vi "sub_register-event-callback.vi"(7 "cmd":enum16{"register", "close"}(ring), 8 "error in":errorcluster, 10 "user param":refnum<vi>[](array[refnum]), 11 "GMapControl":refnum<k24>) -> (0 "error out":errorcluster)   [LabVIEW 2019]
uses:
  dll/GMap.NET.WindowsForms.dll
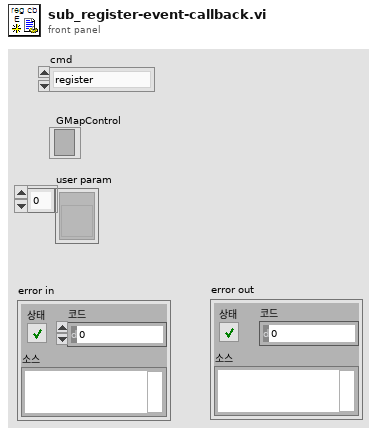
[diagram p1: front panel]
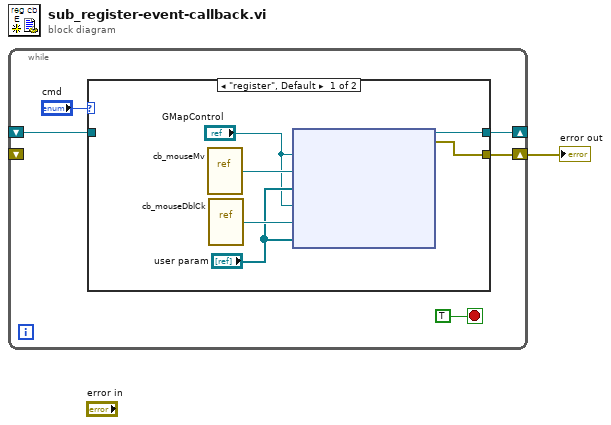
[diagram p0: block diagram]
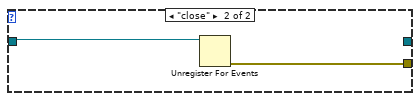
[diagram p2: hidden frame]
diagram:
  n1 = while {
    shift-right: [w3] -> _
    shift-left: _ -> [w4]
    shift-right: [w2] -> w1
    shift-left: _ -> [_]
    stop <- TRUE stop-if-true
    n2 = case shown="\"register\", Default" "cmd" {
      tunnel: w4 -> [_ w14]
      tunnel: [w10 _] -> w3
      tunnel: [w8 w13] -> w2
      frame "register", Default {
        n3 = vi-ref "cb_mouseMv.vi"() -> ("vi reference"=w12:refnum<vi>)
        n4 = vi-ref "cb_mouseDblCk.vi"() -> ("vi reference"=w11:refnum<vi>)
        n5 = node("GMapControl", w12, "user param", "GMapControl", w11, "user param") -> (w10:refnum<k27>, w8:errorcluster)  [unwired: 2 in]
      }
      frame "close" {
        n6 = Unregister For Events(event registration refnum=w14) -> (error out=w13:errorcluster)  [unwired: 1 in]
      }
    }
  }
  "error out" <- w1
